vi "add_vector3.vi"(4 "Vector3":cluster{"x":dbl, "y":dbl, "z":dbl}, 5 "msg in":string) -> (2 "msg out":string)   [LabVIEW 2012]
doc: "Flattens a 3D vector into a string"
uses:
  <userlib>/ROS for LabVIEW Software/ROS/MessageBuilding/std_msgs/subs/float64Scalar.vi
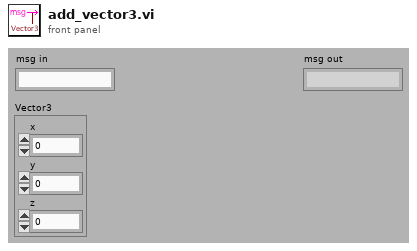
[diagram p1: front panel]
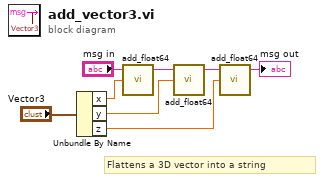
[diagram p0: block diagram]
diagram:
  # "Flattens a 3D vector into a string"
  n1 = Unbundle By Name("Vector3") -> ("x"=w5:dbl, "y"=w4:dbl, "z"=w3:dbl)
  n2 = call-poly <userlib>:"add_float64.vi"("Numeric"=w5, "msg in"="msg in") -> ("msg out"=w8:string)  [unwired: 3 in]
  n3 = call-poly <userlib>:"add_float64.vi"("Numeric"=w4, "msg in"=w8) -> ("msg out"=w7:string)  [unwired: 3 in]
  n4 = call-poly <userlib>:"add_float64.vi"("Numeric"=w3, "msg in"=w7) -> ("msg out"=→"msg out":string)  [unwired: 3 in]
